vi "读取数据处理 (子VI).vi"(0 "Array输入":refnum<vi>, 5 "data out":string, 9 "reference":refnum<vi>) -> (1 "数组":string[](array[string]), 3 "系统编码ST":string, 4 "数组 2":string[](array[string]), 6 "命令编码CN":string, 8 "设备编码MN":string, 10 "密码PW":string, 12 "数据":string, 14 "拆分包及应答Flag":string, 15 "时间QN":string)   [LabVIEW 2016]
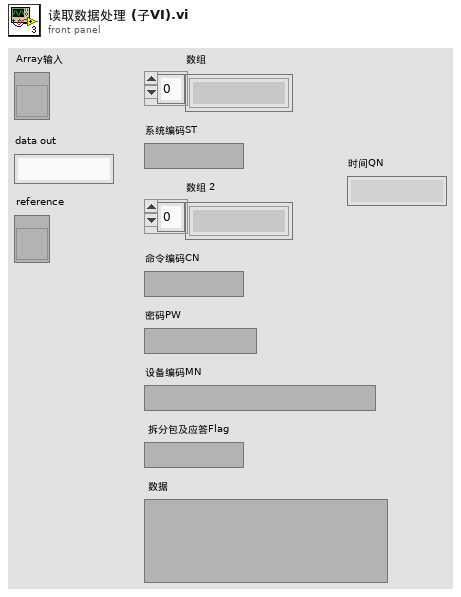
[diagram p1: front panel]
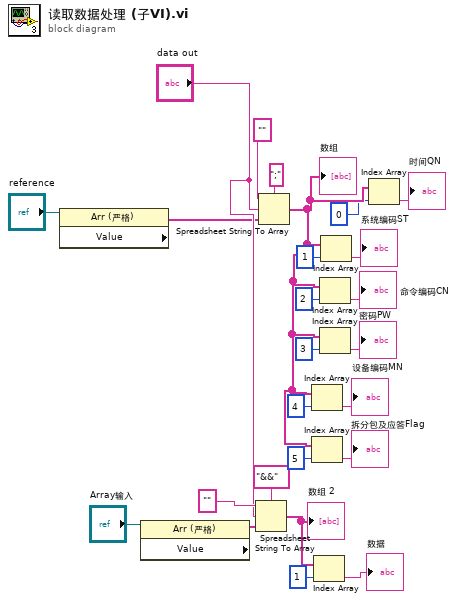
[diagram p0: block diagram]
diagram:
  n1 = property class="Arr (严格)"(reference="reference") -> ("Value"=w8:string[])  [unwired: 1 in, 2 out]
  n2 = property class="Arr (严格)"(reference="Array输入") -> ("Value"=w22:string[])  [unwired: 1 in, 2 out]
  n3 = Spreadsheet String To Array(delimiter (Tab)="&&" ("分隔符(Tab)"), format string="" ("格式字符串"), spreadsheet string="data out", array type (2D Dbl)=w22) -> (array=w23:string[])
  "数组 2" <- w23
  n4 = Spreadsheet String To Array(delimiter (Tab)=";" ("分隔符(Tab)"), format string="" ("格式字符串"), spreadsheet string="data out", array type (2D Dbl)=w8) -> (array=w3:string[])
  "数组" <- w3
  n5 = Index Array(array=w3, index=4 ("索引")) -> (element=→"设备编码MN":string)
  n6 = Index Array(array=w3, index=5 ("索引")) -> (element=→"拆分包及应答Flag":string)
  n7 = Index Array(array=w23, index=1 ("索引")) -> (element=→"数据":string)
  n8 = Index Array(array=w3, index=2 ("索引")) -> (element=→"命令编码CN":string)
  n9 = Index Array(array=w3, index=3 ("索引")) -> (element=→"密码PW":string)
  n10 = Index Array(array=w3, index=1 ("索引")) -> (element=→"系统编码ST":string)
  n11 = Index Array(array=w3, index=0 ("索引")) -> (element=→"时间QN":string)
